vi "array.vi"() -> ()   [LabVIEW 2022 SP3]
panel:
  out "数组":i32[](array[numeric])
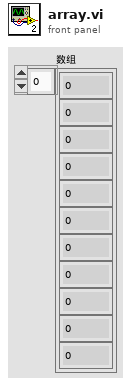
[diagram p1: front panel]
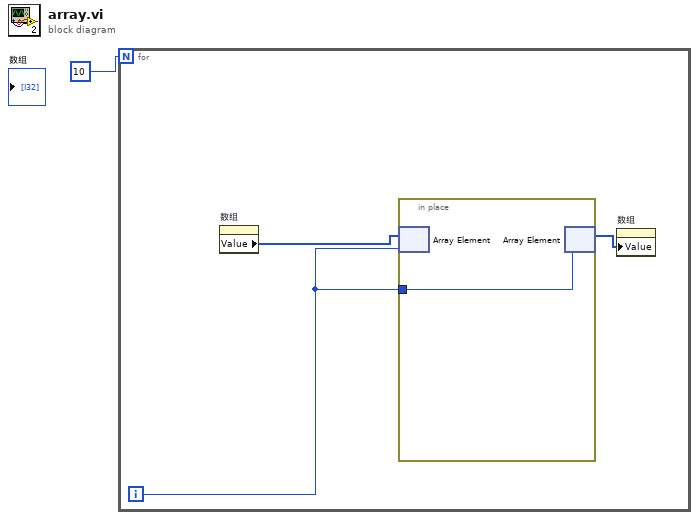
[diagram p0: block diagram]
diagram:
  n1 = for {
    N: 10 -> [_]
    i -> [w2]
    n2 = property on="数组" class="Arr (严格)"() -> ("Value"=w4:i32[])  [unwired: 2 in, 2 out]
    n3 = in-place {
      in-place-border: w2 -> [w5]
      n4 = in-place-array #1(w4, w2) -> ()  [unwired: 1 out]
      n5 = in-place-array #1(w5) -> (w3:i32[])  [unwired: 1 out]
    }
    n6 = property on="数组" class="Arr (严格)"("Value"=w3) -> ()  [unwired: 2 in, 2 out]
  }
